vi "AUTOFOCUS_calculate_noise.vi"(2 "error in":errorcluster, 3 "Ref channel":u16(ring) items=["X signal", "Y signal"]) -> (0 "error out":errorcluster, 1 "Noise":dbl)   [LabVIEW 2015]
uses:
  GLOBAL/Global_FPGA.vi
  <vilib>/gmath/NI_Gmath.lvlib
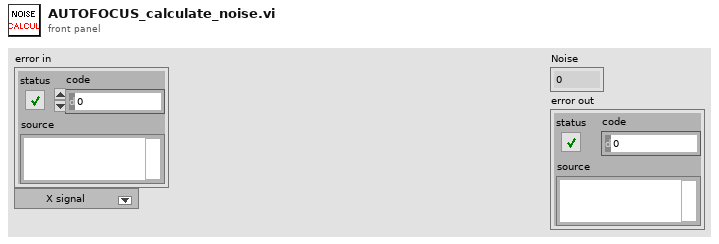
[diagram p1: front panel]
types:
  T1 = cluster{"X":sgl, "Y":sgl, "SUM":sgl, "count":u32}
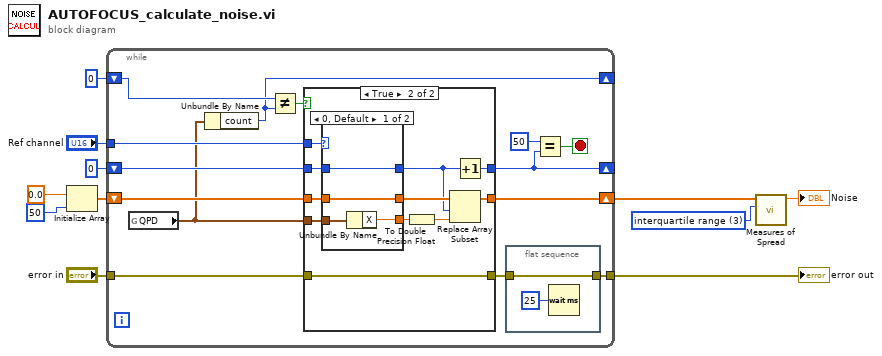
[diagram p0: block diagram]
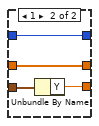
[diagram p3: hidden frame]
diagram:
  w4 = 3 items=["standard deviation", "range", "mean absolute deviation", "interquartile range"] ("type")
  n1 = Initialize Array(0.0 ("element"), 50 ("dimension size")) -> (w10:dbl[])
  n2 = while {
    shift-right: [w22] -> _
    shift-left: 0 -> [w25]
    tunnel: "error in" -> [w12]
    tunnel: [w17] -> w2
    shift-right: [w23] -> w11
    shift-left: w10 -> [w24]
    tunnel: "Ref channel" -> [w19]
    shift-right: [w14] -> _
    shift-left: u32 0 ("count") -> [w15]
    stop <- w20 stop-if-true
    n3 = global read "Global_FPGA.vi" "QPD"() -> (w13:T1)
    n4 = Unbundle By Name(w13) -> ("count"=w14:u32)
    n5 = Not Equal?(x=w15, y=w14) -> (x != y?=w16:bool)
    n6 = case shown="True" w16 {
      tunnel: w12 -> [w30 w31]
      tunnel: [w30 w31] -> w18
      tunnel: w13 -> [_ w40]
      tunnel: w25 -> [w29 w36]
      tunnel: [w29 w41] -> w22
      tunnel: w24 -> [w28 w35]
      tunnel: [w28 w38] -> w23
      tunnel: w19 -> [_ w32]
      frame False {
      }
      frame True {
        n7 = case shown="0, Default" w32 {
          tunnel: w40 -> [w43 w49]
          tunnel: [w42 w48] -> w39
          tunnel: w36 -> [w45 w46]
          tunnel: w35 -> [w44 w47]
          tunnel: [w44 w47] -> w34
          tunnel: [w45 w46] -> w33
          frame 0, Default {
            n8 = Unbundle By Name(w43) -> ("X"=w42:sgl)
          }
          frame 1 {
            n9 = Unbundle By Name(w49) -> ("Y"=w48:sgl)
          }
        }
        n10 = To Double Precision Float(number=w39) -> (double precision float=w37:dbl)
        n11 = Replace Array Subset(array=w34, new element=w37, index=w33) -> (w38:dbl[])
        n12 = Increment(x=w33) -> (x+1=w41:i32)
      }
    }
    n13 = flat-sequence {
      tunnel: w18 -> [w27]
      tunnel: [w27] -> w17
      frame #0 {
        n14 = Wait (ms)(milliseconds to wait=u32 25) -> ()  [unwired: 1 out]
      }
    }
    n15 = Equal?(x=50, y=w22) -> (x = y?=w20:bool)
  }
  "error out" <- w2
  n16 = call <vilib>:"Measures of Spread.vi"("type"=w4, "x array"=w11) -> ("spread value"=→"Noise":dbl)  [unwired: 8 in, 1 out]
